vi "Analog Read.vi"() -> ()   [LabVIEW 2017]
uses:
  <vilib>/Instr/_visa.llb/VISA Configure Serial Port (Instr).vi
panel:
  out "pph":u8(slide) scale=0.0..1000.0
  in  "USB Serial Port":refnum<visa-resource-name>
  out "Waveform Chart":dbl(graph)
  out "Table":string[][](table)
  out "Pressure Value of Gas":string
  in  "Home Button":bool=TRUE
  in  "Stop":bool
  out "Result":string
  in  "Play Button":bool=TRUE
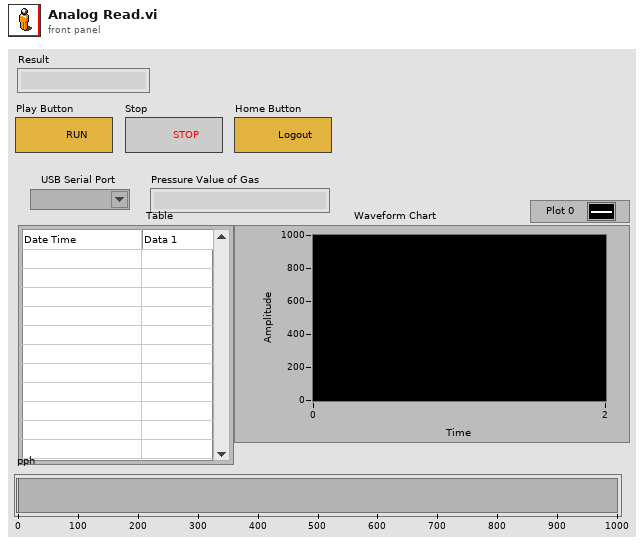
[diagram p1: front panel]
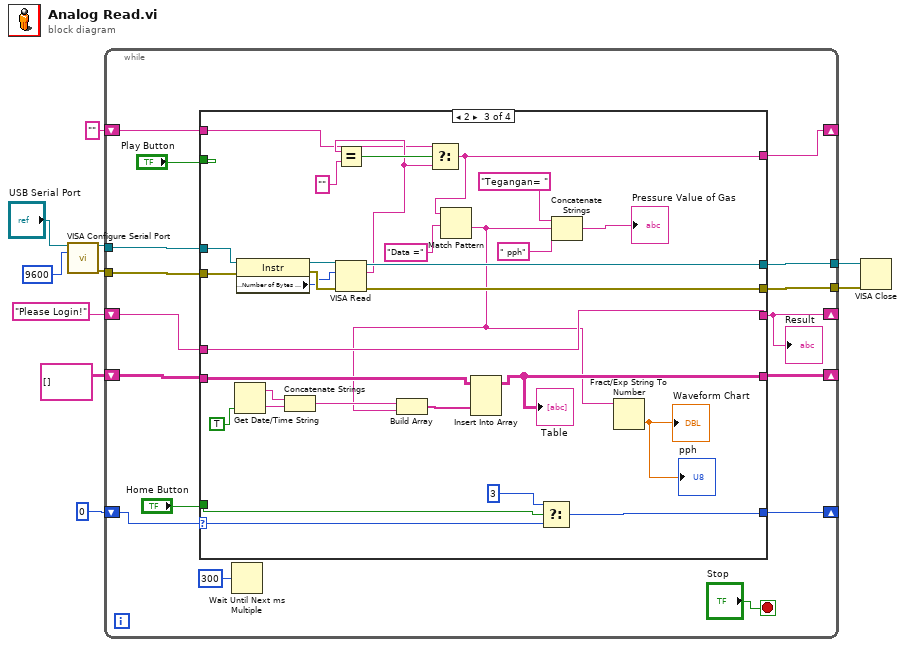
[diagram p0: block diagram]
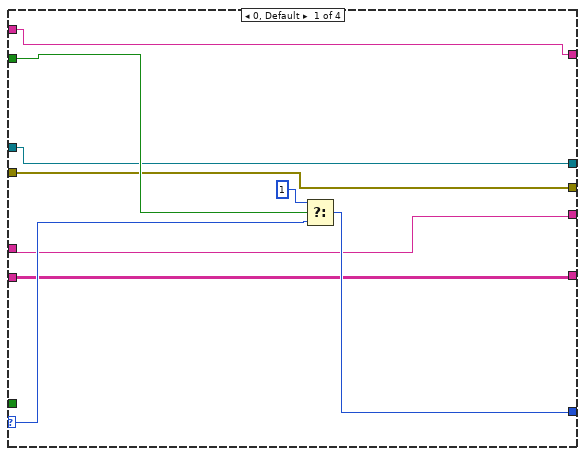
[diagram p2: hidden frame]
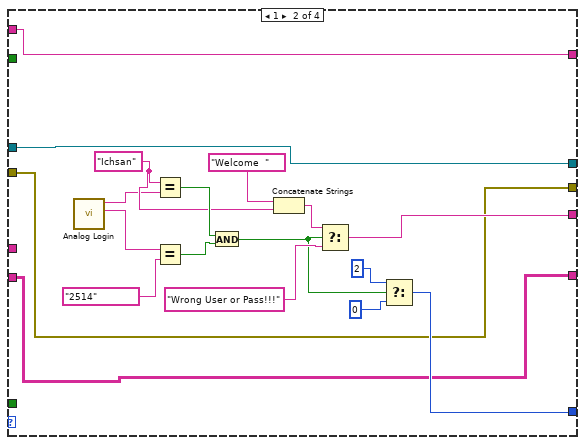
[diagram p3: hidden frame]
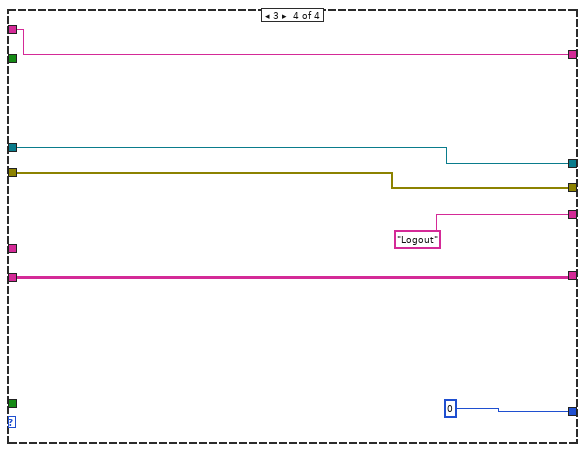
[diagram p4: hidden frame]
diagram:
  n1 = call-poly "VISA Configure Serial Port"("VISA resource name"="USB Serial Port", "baud rate (9600)"=u32 9600 ("byte count")) -> ("VISA resource name out"=w3:refnum<visa-resource-name>, "error out"=w4:errorcluster)  [unwired: 12 in]
  n2 = while {
    shift-right: [w26] -> _
    shift-left: 0 -> [w22]
    shift-right: [w21] -> _
    shift-left: "Please Login!" ("String") -> [w20]
    tunnel: w3 -> [w19]
    tunnel: w4 -> [w18]
    tunnel: [w17] -> w8
    tunnel: [w16] -> w7
    shift-right: [w14] -> _
    shift-left: string[][] [] -> [w13]
    shift-right: [w11] -> _
    shift-left: "" -> [w12]
    stop <- "Stop" stop-if-true
    n3 = case shown="2" w22 {
      selector: w22 -> [w33 _ w81 _]
      tunnel: [w35 w53 w83 0] -> w26
      tunnel: "Play Button" -> [w34 _ _ _]
      tunnel: "Home Button" -> [_ _ w80 _]
      tunnel: [w31 w42 w79 "Logout" ("String")] -> w21
      tunnel: w20 -> [w31 _ w79 _]
      tunnel: w19 -> [w30 w39 w78 w87]
      tunnel: w18 -> [w29 w38 w77 w86]
      tunnel: [w29 w38 w74 w86] -> w17
      tunnel: [w30 w39 w73 w87] -> w16
      tunnel: [w28 w37 w64 w85] -> w14
      tunnel: w13 -> [w28 w37 w65 w85]
      tunnel: w12 -> [w27 w36 w55 w84]
      tunnel: [w27 w36 w54 w84] -> w11
      frame 0, Default {
        n4 = Select(t=1, s=w34, f=w33) -> (s? t:f=w35:i32)
      }
      frame 1 {
        w43 = "Ichsan"
        n5 = call "Analog Login.vi"() -> ("Password 2"=w40:string, "User Name 2"=w41:string)  [unwired: 9 in, 1 out]
        n6 = Equal?(x=w43, y=w41) -> (x = y?=w46:bool)
        n7 = Equal?(x=w40, y="2514") -> (x = y?=w45:bool)
        n8 = And(x=w46, y=w45) -> (x .and. y?=w47:bool)
        n9 = Concatenate Strings("Welcome  ", w43) -> (w50:string)
        n10 = Select(t=w50, s=w47, f="Wrong User or Pass!!!") -> (s? t:f=w42:string)
        n11 = Select(t=2, s=w47, f=0) -> (s? t:f=w53:i32)
      }
      frame 2 {
        n12 = Get Date/Time String(want seconds? (F)=TRUE) -> (date string=w67:string, time string=w66:string)  [unwired: 2 in]
        n13 = property class="Instr"(reference=w78, error in=w77) -> (reference out=w76:refnum<visa-resource-name>, error out=w75:errorcluster, "Serial Settings:Number of Bytes at Serial Port"=w63:u32)
        n14 = Concatenate Strings(w67, w66) -> (w62:string)
        n15 = VISA Read(VISA resource name=w76, byte count=w63, error in (no error)=w75) -> (VISA resource name out=w73:refnum<visa-resource-name>, read buffer=w56:string, error out=w74:errorcluster)  [unwired: 1 out]
        n16 = Equal?(x=w56, y="" ("regular expression")) -> (x = y?=w57:bool)
        n17 = Select(t=w55, s=w57, f=w56) -> (s? t:f=w54:string)
        n18 = Match Pattern(string=w54, regular expression="Data =") -> (after substring=w60:string)  [unwired: 1 in, 3 out]
        n19 = Build Array(w62, w60) -> (w61:string[])
        n20 = Insert Into Array(array=w65, new element=w61) -> (w64:string[][])  [unwired: 2 in]
        "Table" <- w64
        n21 = Select(t=3, s=w80, f=w81) -> (s? t:f=w83:i32)
        n22 = Concatenate Strings("Tegangan= " ("string"), w60, " pph" ("string")) -> (→"Pressure Value of Gas":string)
        n23 = Fract/Exp String To Number(string=w60) -> (number=→"Waveform Chart" →"pph":dbl)  [unwired: 3 in, 1 out]
      }
      frame 3 {
      }
    }
    "Result" <- w21
    n24 = Wait Until Next ms Multiple(millisecond multiple=u32 300) -> ()  [unwired: 1 out]
  }
  n25 = VISA Close(VISA resource name=w7, error in (no error)=w8) -> ()  [unwired: 1 out]
